vi "Read TCS string.vi"(8 "error in (no error)":errorcluster, 11 "Telemetry in":refnum<class "Telemetry.lvclass">) -> (0 "error out":errorcluster, 2 "TCS string":string, 3 "Telemetry out":refnum<class "Telemetry.lvclass">)   [LabVIEW 2018, in "Telemetry.lvclass"]
uses:
  Telemetry.lvclass
  Telemetry.lvclass/Telemetry.ctl
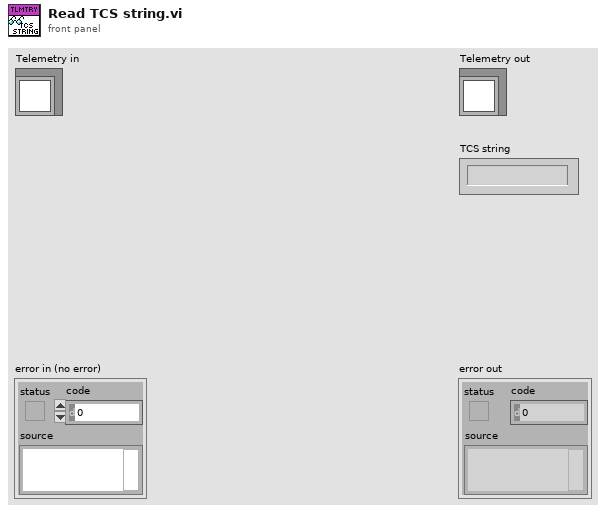
[diagram p1: front panel]
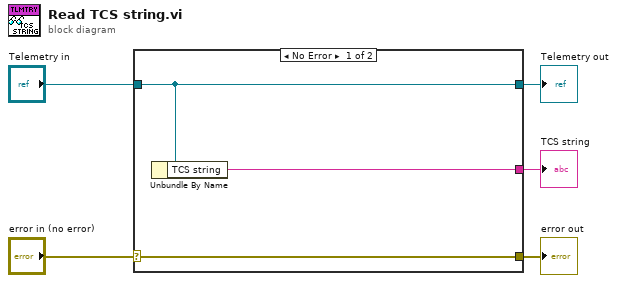
[diagram p0: block diagram]
diagram:
  n1 = case shown="No Error" "error in (no error)" {
    selector: "error in (no error)" -> [w8 w9]
    tunnel: [w8 w9] -> w4
    tunnel: [w7 w10] -> w2
    tunnel: "Telemetry in" -> [w7 w10]
    tunnel: [w6 _] -> w1
    frame No Error {
      n2 = Unbundle By Name(w7) -> ("TCS string"=w6:string)
    }
    frame Error {
    }
  }
  "error out" <- w4
  "Telemetry out" <- w2
  "TCS string" <- w1
